vi "Read Counter Input PWM Module.vi"   [LabVIEW 2020, in "Scan Engine Scripting.lvlib"]
doc: "Returns the channel settings of a counter input PWM module that can be edited and then used to create a new module instance to set into a slot."
uses:
  Scan Engine Scripting.lvlib
  Modules/NI 9423/NI 9423.lvclass
  Modules/NI 9437/NI 9437.lvclass
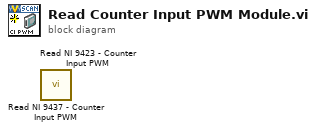
[diagram p0: block diagram]
diagram:
  n1 = call "Read NI 9437 - Counter Input PWM.vi"() -> ()  [unwired: 9 in, 3 out]
  n2 = call "Read NI 9423 - Counter Input PWM.vi"() -> ()  [unwired: 9 in, 3 out]
